vi "ejemplo_graph.vi"() -> ()   [LabVIEW 2020]
panel:
  out "Waveform Graph":dynamicdata(graph)
  out "Numeric":dbl
  in  "stop":bool
  out "Boolean":bool
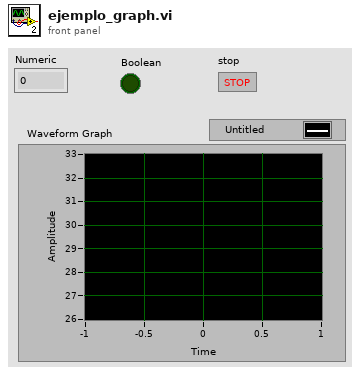
[diagram p1: front panel]
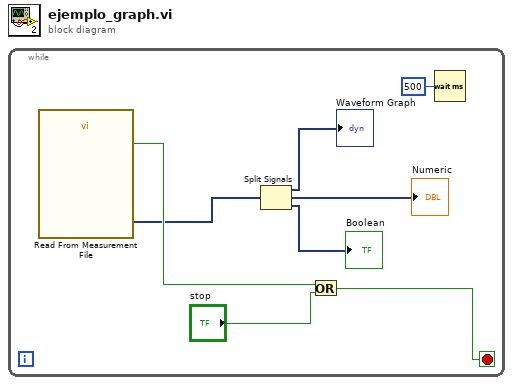
[diagram p0: block diagram]
diagram:
  n1 = while {
    stop <- w6 stop-if-true
    n2 = call "Read From Measurement File"() -> ("Signals"=w4:dynamicdata, "EOF?"=w7:bool)  [unwired: 6 in, 4 out]
    n3 = Split Signals(w4) -> (→"Waveform Graph":dynamicdata, →"Numeric":dynamicdata, →"Boolean":dynamicdata)  [unwired: 3 in]
    n4 = Or(x=w7, y="stop") -> (x .or. y?=w6:bool)
    n5 = Wait (ms)(milliseconds to wait=u32 500) -> ()  [unwired: 1 out]
  }
